vi "BotSpeak_System.vi"(2 "Values sent":i16[](array[numeric]), 3 "Variable In":string="power", 4 "Bot Settings":T1) -> (1 "Bot Settings":T1)   [LabVIEW 2014]
doc: "Calls customized system call on \"variable in\" and assigns \"values sent\" within the function"
uses:
  <userlib>/BotSpeak/VIs/Direct/BotSpeak_Control.ctl
panel:
  out "response":string
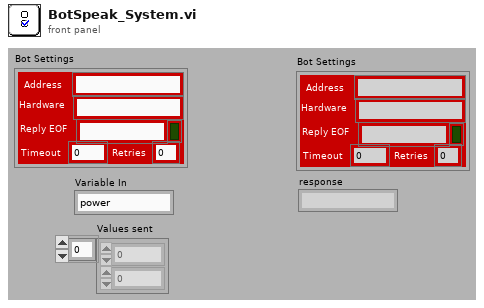
[diagram p1: front panel]
types:
  T1 = typedef "BotSpeak_Control.ctl" = cluster{"Address":string, "Reply EOF":string, "Hardware":string, "Retries":i8, "Timeout":i32, "Open?":bool}
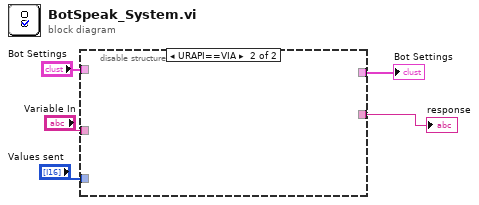
[diagram p0: block diagram]
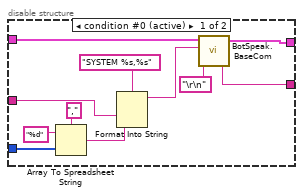
[diagram p2: hidden frame]
diagram:
  n1 = disable-structure shown="URAPI==VIA" {
    disable-tunnel: "Bot Settings" -> [w15 _]
    disable-tunnel: [w14 _] -> w4
    disable-tunnel: [w12 _] -> w3
    disable-tunnel: "Values sent" -> [w11 _]
    disable-tunnel: "Variable In" -> [w6 _]
    frame condition #0 (active) {
      n2 = Array To Spreadsheet String(delimiter (Tab)=",", array=w11, 3:"%d" ("format string")) -> (spreadsheet string=w8:string)
      n3 = Format Into String(format string="SYSTEM %s,%s" ("command"), w6, w8) -> (resulting string=w16:string)  [unwired: 2 in, 1 out]
      n4 = call <userlib>:"BotSpeak.BaseCom.vi"("Termination"="\r\n", "command"=w16, "Bot Settings in"=w15) -> ("response"=w12:string, "Bot Settings out"=w14:T1)  [unwired: 2 in]
    }
    frame condition #1 {
    }
  }
  "Bot Settings" <- w4
  "response" <- w3
